vi "CalculateAreaScanVelocity.vi"(5 "error in (no error)":errorcluster) -> (19 "error out":errorcluster)   [LabVIEW 2014]
doc: "This VI calculates the velocity that has to be specified at a area scan routine definition.\nthe user can specify the desired \"step size\" and the velocity (either the scan axis velocity [sinusodial] or the radial velocity [spiral]) is calculated from the frequency and the selected routine type."
panel:
  in  "Target type":i32
  in  "Calculate":bool
  out "Resulting Velocity":dbl format="%.4f"
  in  "Frequency":dbl format="%.3f"
  in  "Desired Step size of scan axis":dbl=0.1 format="%.4f"
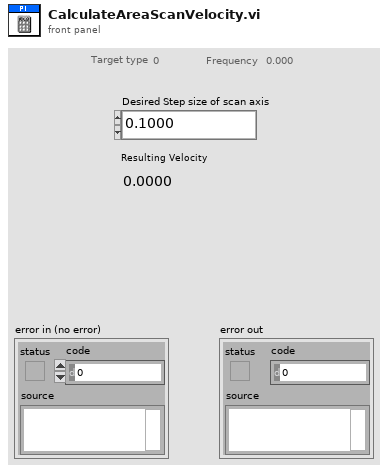
[diagram p1: front panel]
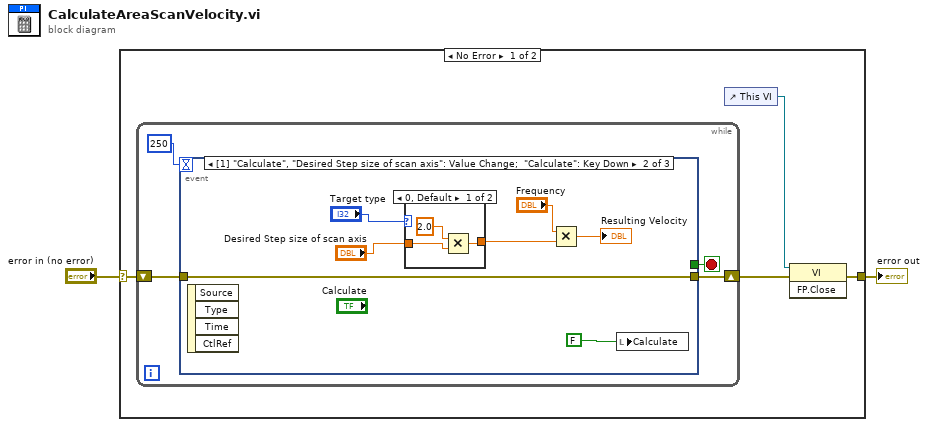
[diagram p0: block diagram]
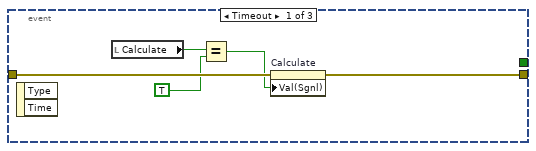
[diagram p2: hidden frame]
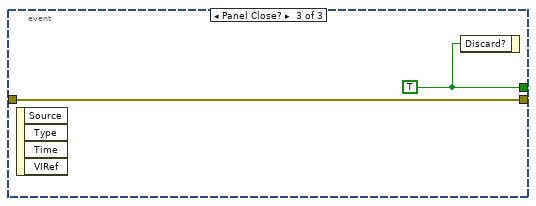
[diagram p4: hidden frame]
diagram:
  n1 = case shown="No Error" "error in (no error)" {
    selector: "error in (no error)" -> [w6 w29]
    tunnel: [w3 w29] -> w1
    frame No Error {
      n2 = while {
        shift-right: [w9] -> w4
        shift-left: w6 -> [w10]
        stop <- w8 stop-if-true
        n3 = event shown="[1] \"Calculate\", \"Desired Step size of scan axis\": Value Change;  \"Calculate\": Key Down" {
          selector: _ -> [_ _ _]
          dyn-events: _ -> [_ _ _]
          timeout: 250 ("Numeric") -> [_ _ _]
          tunnel: w10 -> [w14 w21 w28]
          tunnel: [w13 w21 w28] -> w9
          tunnel: [_ _ w27] -> w8
          event Timeout {
            n4 = event-data() -> ()  [unwired: 3 out]
            n5 = local read "Calculate"() -> (w15:bool)
            n6 = Equal?(x=w15, y=TRUE) -> (x = y?=w11:bool)
            n7 = property on="Calculate" class="Bool (strict)"(error in=w14, "Val(Sgnl)"=w11) -> (error out=w13:errorcluster)  [unwired: 1 in, 1 out]
          }
          event "Calculate", "Desired Step size of scan axis": Value Change; "Calculate": Key Down {
            n8 = event-data() -> ()  [unwired: 5 out]
            n9 = case shown="0, Default" "Target type" {
              tunnel: "Desired Step size of scan axis" -> [w24 w26]
              tunnel: [w23 w26] -> w17
              frame 0, Default {
                n10 = Multiply(x=2.0 ("y"), y=w24) -> (x*y=w23:dbl)
              }
              frame 1 {
              }
            }
            n11 = Multiply(x="Frequency", y=w17) -> (x*y=→"Resulting Velocity":dbl)
            n12 = local write "Calculate"(FALSE) -> ()
          }
          event Panel Close? {
            w27 = TRUE
            n13 = event-data() -> ()  [unwired: 5 out]
            n14 = event-data("Discard?"=w27) -> ()  [unwired: 1 in, 1 out]
          }
        }
      }
      n15 = control-ref of="This VI"() -> (w5:refnum<vi>)
      n16 = invoke class="VI" method="FP.Close"(reference=w5, error in=w4) -> (error out=w3:errorcluster)  [unwired: 1 in, 2 out]
    }
    frame Error {
    }
  }
  "error out" <- w1
